vi "keeponly_msb_I16.vi"(11 "x":i16 format="%b") -> (3 "y":u16)   [LabVIEW 2018, in "posit.lvlib"]
uses:
  posit.lvlib
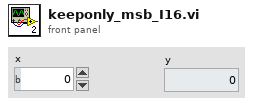
[diagram p1: front panel]
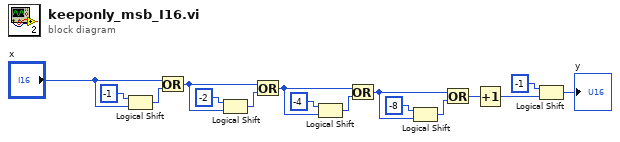
[diagram p0: block diagram]
diagram:
  n1 = Logical Shift(y=i16 -1 ("x"), x="x") -> (x << y=w1:i16)
  n2 = Or(x="x", y=w1) -> (x .or. y?=w5:i16)
  n3 = Logical Shift(y=i16 -2 ("x"), x=w5) -> (x << y=w6:i16)
  n4 = Or(x=w5, y=w6) -> (x .or. y?=w9:i16)
  n5 = Logical Shift(y=i16 -4 ("x"), x=w9) -> (x << y=w8:i16)
  n6 = Or(x=w9, y=w8) -> (x .or. y?=w12:i16)
  n7 = Logical Shift(y=i16 -8 ("x"), x=w12) -> (x << y=w11:i16)
  n8 = Or(x=w12, y=w11) -> (x .or. y?=w13:i16)
  n9 = Increment(x=w13) -> (x+1=w15:i16)
  n10 = Logical Shift(y=i16 -1 ("x"), x=w15) -> (x << y=→"y":i16)
